vi "first_pass.vi"() -> ()   [LabVIEW 2016]
panel:
  in  "?":bool
  in  "?":bool
  in  "Confirm Start":bool
  out "Nozzle":cluster{"X":dbl, "Y":dbl}[](graph)
  out "Pre-Combustion Chamber":cluster{"X":dbl, "Y":dbl}[](graph)
  out "Battery Voltage":u8(slide) scale=0.0..100.0
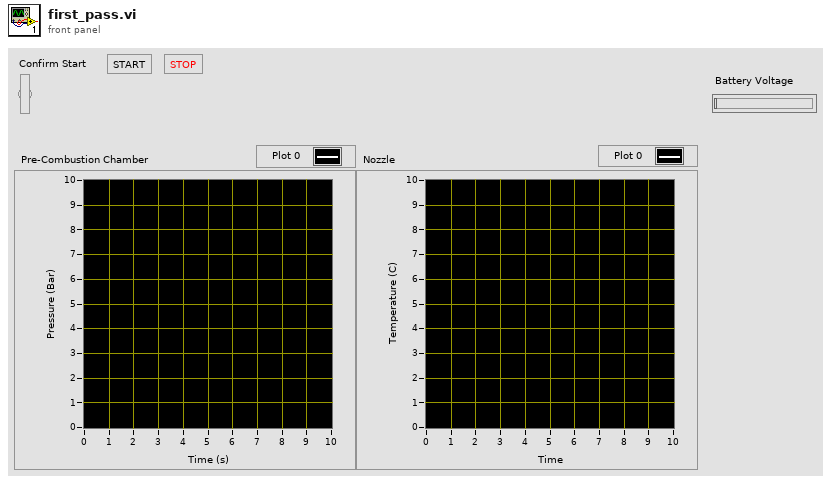
[diagram p1: front panel]
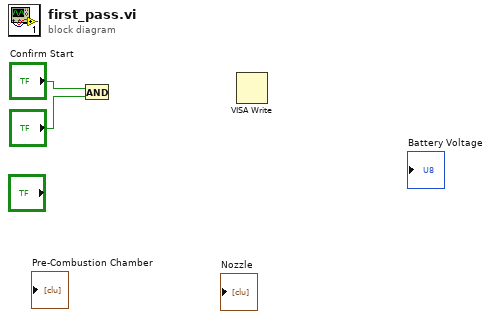
[diagram p0: block diagram]
diagram:
  n1 = And(x="Confirm Start", y="?") -> ()  [unwired: 1 out]
  n2 = VISA Write() -> ()  [unwired: 3 in, 3 out]
